vi "tempcrap2.vi"   [LabVIEW 2013]
types:
  T1 = typedef "LVRectTypeDef.ctl" = cluster{"Left":i16, "Top":i16, "Right":i16, "Bottom":i16}
  T2 = cluster{"Xpixels":i32, "Vx-min ref":dbl, "Vx-max ref":dbl, "P":dbl, "Ypixels":i32, "Vy-min ref":dbl, "Vy-max ref":dbl, "srate":sgl, "sAOxy":i32, "timeout":dbl, "type":string, "date":string, "time":string, "Colormap":u16, "Drawing Mode":u16, "Scanning Mode":u16, "square pixels":bool, "square matrix":bool, "Xpixels Img":i32, "Vx-min Img":dbl, "VX-max Img":dbl, "Ypixels Img":i32, "Vy-min Img":dbl, "Vy-max Img ":dbl, "Angle Img":dbl, "autoshutter":bool, "finite":bool, "cont":bool, "wavdet":bool, "measpoints":i32, "avpp":i32, "bufferAO":i32, "bufferAI":i32, "CH1":bool, "CH2":bool, "X":bool, "Y":bool, "Ip":bool, "Vp":bool, "starttick":u32, "waveform":path, "Vx-ref":dbl, "Vy-ref":dbl, "refreshrate":dbl, "refreshbuffer":i32, "tt_cycles":i32, "motorref":refnum<k7>, "mirrorswitch":refnum<k7>, "sample mode":i32, "maxbufferAI":i32, "sampletreshold":dbl, "srateAODO":sgl, "bin":sgl, "Pel":sgl, "Angle draw":dbl, "srate Img":sgl, "ROIimg_plotbounds":T1}
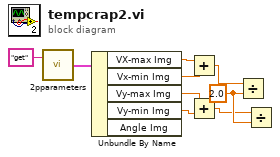
[diagram p0: block diagram]
diagram:
  w2 = 2.0 ("y")
  n1 = call "2pparameters.vi"("command"="get") -> ("Params out"=w7:T2)  [unwired: 1 in]
  n2 = Unbundle By Name(w7) -> ("VX-max Img"=w8:dbl, "Vx-min Img"=w9:dbl, "Vy-max Img"=w4:dbl, "Vy-min Img"=w3:dbl)  [unwired: 1 out]
  n3 = Add(x=w8, y=w9) -> (x+y=w5:dbl)
  n4 = Add(x=w4, y=w3) -> (x+y=w1:dbl)
  n5 = Divide(x=w5, y=w2) -> ()  [unwired: 1 out]
  n6 = Divide(x=w1, y=w2) -> ()  [unwired: 1 out]
